vi "Move one step in grid.vi"(10 "Tail Positions":T1, 11 "Head Position":T1) -> (3 "New Tail Position":T1)   [LabVIEW 2021]
uses:
  Positions.ctl
panel:
  out "number":u32
  out "x = y? 2":bool
  out "x = y?":bool
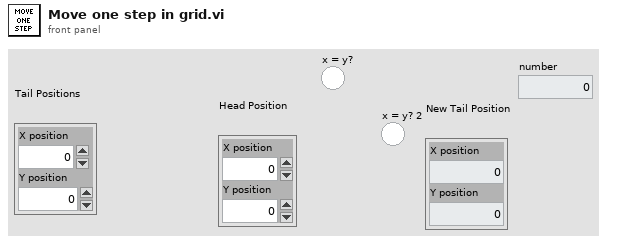
[diagram p1: front panel]
types:
  T1 = typedef "Positions.ctl" = cluster{"X position":i32, "Y position":i32}
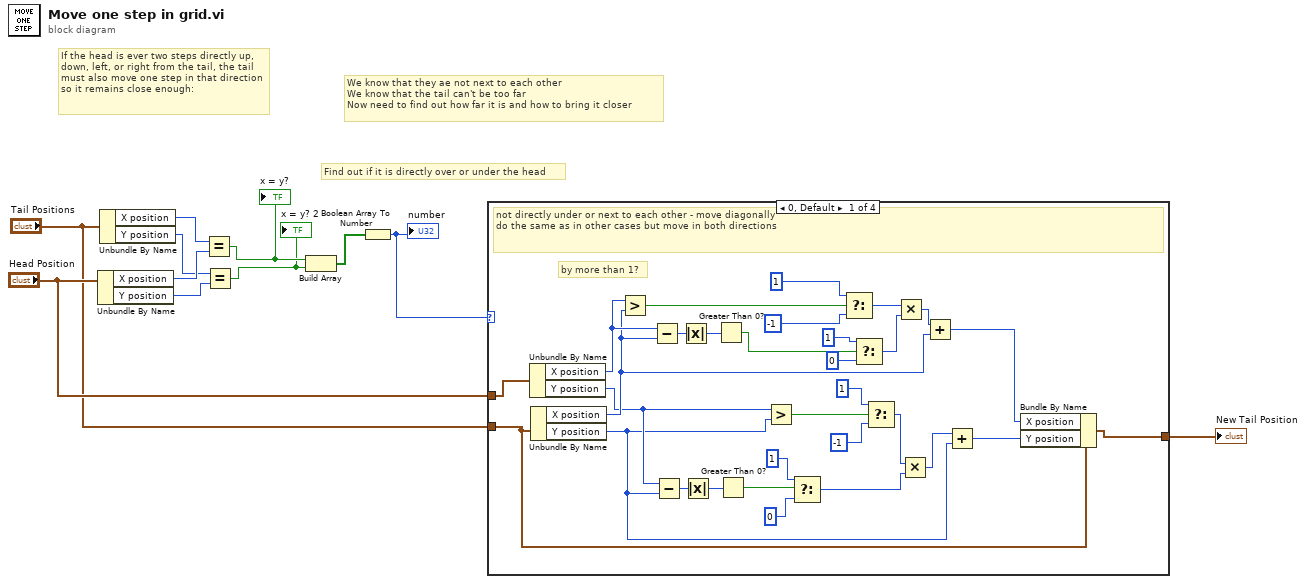
[diagram p0: block diagram]
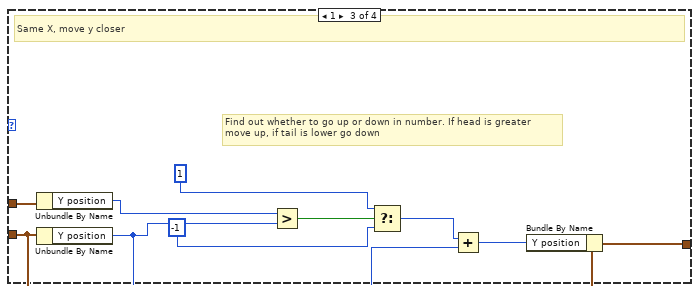
[diagram p3: hidden frame]
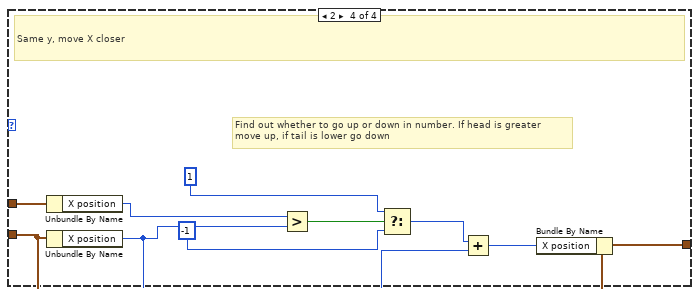
[diagram p4: hidden frame]
diagram:
  # "Find out if it is directly over or under the head"
  # "We know that they ae not next to each other\nWe know that the tail can't be too far\nNow need to find out how far it is and how to bring it closer"
  # "If the head is ever two steps directly up, down, left, or right from the tail, the tail must also move one step in that direction so it remains close enough:"
  n1 = Unbundle By Name("Head Position") -> ("X position"=w10:i32, "Y position"=w8:i32)
  n2 = Unbundle By Name("Tail Positions") -> ("X position"=w11:i32, "Y position"=w9:i32)
  n3 = Equal?(x=w11, y=w10) -> (x = y?=w7:bool)
  "x = y?" <- w7
  n4 = Equal?(x=w9, y=w8) -> (x = y?=w6:bool)
  "x = y? 2" <- w6
  n5 = Build Array(w7, w6) -> (w5:bool[])
  n6 = Boolean Array To Number(Boolean array=w5) -> (number=w4:u32)
  "number" <- w4
  n7 = case shown="0, Default" w4 {
    tunnel: "Head Position" -> [w38 _ w53 w56]
    tunnel: "Tail Positions" -> [w37 w43 w52 w55]
    tunnel: [w32 w43 w44 w54] -> w1
    frame 0, Default {
      # "by more than 1?"
      # "not directly under or next to each other - move diagonally\ndo the same as in other cases but move in both directions"
      n8 = Unbundle By Name(w38) -> ("X position"=w31:i32, "Y position"=w19:i32)
      n9 = Unbundle By Name(w37) -> ("X position"=w30:i32, "Y position"=w18:i32)
      n10 = Greater?(x=w31, y=w30) -> (0:w36:bool)
      n11 = Subtract(x=w31, y=w30) -> (x-y=w29:i32)
      n12 = Subtract(x=w19, y=w18) -> (x-y=w21:i32)
      n13 = Absolute Value(x=w29) -> (abs(x)=w28:i32)
      n14 = Absolute Value(x=w21) -> (abs(x)=w20:i32)
      n15 = Greater Than 0?(x=w28) -> (x > 0?=w26:bool)
      n16 = Greater Than 0?(x=w20) -> (x > 0?=w15:bool)
      n17 = Greater?(x=w19, y=w18) -> (0:w42:bool)
      n18 = Select(t=1 ("Y position"), s=w15, f=0) -> (s? t:f=w14:i32)
      n19 = Select(t=1 ("Y position"), s=w36, f=-1 ("Y position")) -> (s? t:f=w27:i32)
      n20 = Select(t=1 ("Y position"), s=w26, f=0) -> (s? t:f=w23:i32)
      n21 = Select(t=1 ("Y position"), s=w42, f=-1 ("Y position")) -> (s? t:f=w13:i32)
      n22 = Multiply(x=w27, y=w23) -> (x*y=w22:i32)
      n23 = Multiply(x=w13, y=w14) -> (x*y=w12:i32)
      n24 = Add(x=w22, y=w30) -> (x+y=w33:i32)
      n25 = Add(x=w12, y=w18) -> (x+y=w39:i32)
      n26 = Bundle By Name(cluster=w37, "X position"=w33, "Y position"=w39) -> (w32:T1)
    }
    frame 3 {
      # "They overlap. This should not happen"
    }
    frame 1 {
      # "Find out whether to go up or down in number. If head is greater\nmove up, if tail is lower go down"
      # "Same X, move y closer"
      n27 = Unbundle By Name(w53) -> ("Y position"=w51:i32)
      n28 = Unbundle By Name(w52) -> ("Y position"=w46:i32)
      n29 = Greater?(x=w51, y=w46) -> (0:w50:bool)
      n30 = Select(t=1 ("Y position"), s=w50, f=-1 ("Y position")) -> (s? t:f=w47:i32)
      n31 = Add(x=w47, y=w46) -> (x+y=w45:i32)
      n32 = Bundle By Name(cluster=w52, "Y position"=w45) -> (w44:T1)
    }
    frame 2 {
      # "Find out whether to go up or down in number. If head is greater\nmove up, if tail is lower go down"
      # "Same y, move X closer"
      n33 = Unbundle By Name(w56) -> ("X position"=w63:i32)
      n34 = Unbundle By Name(w55) -> ("X position"=w58:i32)
      n35 = Greater?(x=w63, y=w58) -> (0:w62:bool)
      n36 = Select(t=1 ("Y position"), s=w62, f=-1 ("Y position")) -> (s? t:f=w59:i32)
      n37 = Add(x=w59, y=w58) -> (x+y=w57:i32)
      n38 = Bundle By Name(cluster=w55, "X position"=w57) -> (w54:T1)
    }
  }
  "New Tail Position" <- w1
